vi "Arduino End Comms.vi"(1 "Resource index":i32, 2 "VISA resource name":refnum<visa-resource-name>) -> (0 "Error":errorcluster, 3 "Arduino VISA config & resource":T1={"baud rate (bps)"=276000, "timeout (ms)"=12000, "data bits"=8, "parity"=enum."None", "stop bits (10: 1 bit)"=10, "flow control"=0, "termination char (hex)"=10, "Enable Termination Char"=FALSE, "byte count"=12, "Resource locked?"=FALSE, "VISA resource name"=""} {"termination char (hex)" format="%02x"; "stop bits (10: 1 bit)" items=["1.0"=10, "1.5"=15, "2.0"=20]; "flow control" items=["None", "XON/XOFF", "RTS/CTS", "XON/XOFF & RTS/CTS", "DTR/DSR", "XON/XOFF & DTR/DSR"]})   [LabVIEW 2022 SP3]
uses:
  ctls_and_globals/Arduino Config & resource typedef.ctl
  ctls_and_globals/Arduino Global.vi
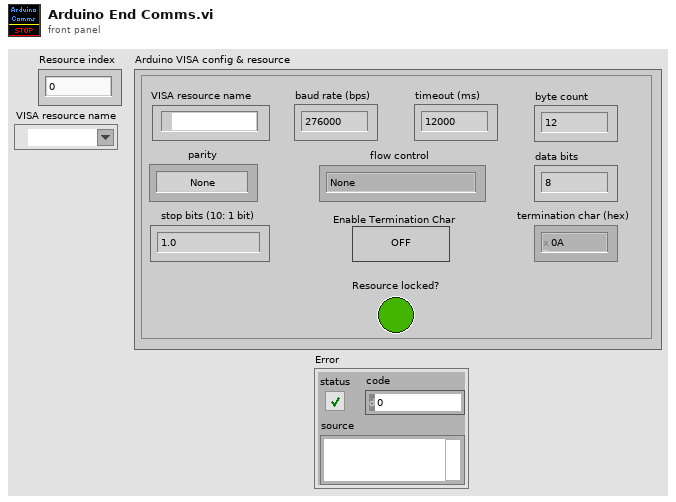
[diagram p1: front panel]
types:
  T1 = typedef "Arduino Config & resource typedef.ctl" = cluster{"baud rate (bps)":u32, "timeout (ms)":u32, "data bits":u16, "parity":enum16{"None", "Odd", "Even", "Mark", "Space"}, "stop bits (10: 1 bit)":u16, "flow control":u16, "termination char (hex)":u8, "Enable Termination Char":bool, "byte count":u32, "Resource locked?":bool, "VISA resource name":refnum<visa-resource-name>}
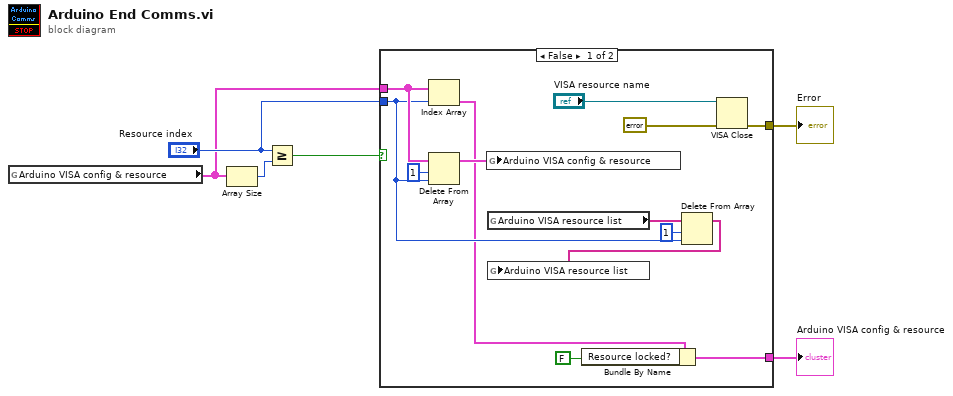
[diagram p0: block diagram]
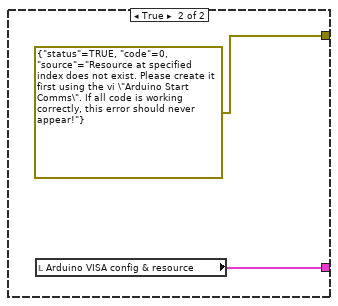
[diagram p2: hidden frame]
diagram:
  n1 = global read "Arduino Global.vi" "Arduino VISA config & resource"() -> (w2:T1[])
  n2 = Array Size(array=w2) -> (size(s)=w6:i32)
  n3 = Greater Or Equal?(x="Resource index", y=w6) -> (x >= y?=w5:bool)
  n4 = case shown="False" w5 {
    tunnel: [w19 errorcluster {"status"=TRUE, "code"=0, "source"="Resource at specified index does not exist. Please create it first using the vi \"Arduino Start Comms\". If all code is working correctly, this error should never appear!"} ("error out")] -> w4
    tunnel: "Resource index" -> [w11 _]
    tunnel: w2 -> [w18 _]
    tunnel: [w14 w20] -> w1
    frame False {
      n5 = Index Array(array=w18, index=w11) -> (element=w9:T1)
      n6 = Delete From Array(array=w18, length=1, index=w11) -> (array with subset deleted=w16:T1[])  [unwired: 1 out]
      n7 = global write "Arduino Global.vi" "Arduino VISA config & resource"(w16) -> ()
      n8 = global read "Arduino Global.vi" "Arduino VISA resource list"() -> (w12:string[])
      n9 = Bundle By Name(cluster=w9, "Resource locked?"=FALSE) -> (w14:T1)
      n10 = Delete From Array(array=w12, length=1, index=w11) -> (array with subset deleted=w10:string[])  [unwired: 1 out]
      n11 = global write "Arduino Global.vi" "Arduino VISA resource list"(w10) -> ()
      n12 = VISA Close(VISA resource name="VISA resource name", error in (no error)=errorcluster {"status"=FALSE, "code"=0, "source"=""}) -> (error out=w19:errorcluster)
    }
    frame True {
      n13 = local read "Arduino VISA config & resource"() -> (w20:T1)
    }
  }
  "Arduino VISA config & resource" <- w1
  "Error" <- w4
